vi "Gear.vi"(10 "Gear1?":bool, 11 "Gear0?":bool) -> ()   [LabVIEW 2016]
uses:
  <vilib>/Rock Robotics/WPI/Solenoid/WPI_SolenoidValue.ctl
  <vilib>/Rock Robotics/WPI/Solenoid/WPI_SolenoidSetEnum.vi
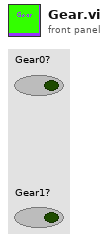
[diagram p1: front panel]
types:
  T1 = typedef "WPI_SolenoidValue.ctl" = enum16{"Off", "On", "Forward", "Reverse"}
  T2 = typedef "WPI_SolenoidDevRef.ctl" = cluster{"DevStatus":errorcluster, "Pneumatics Control Module":u8, "Forward Solenoid Channel":T3, "Reverse Solenoid Channel":T3}
  T3 = typedef "WPI_SolenoidChannel.ctl" = enum8{"Solenoid 0", "Solenoid 1", "Solenoid 2", "Solenoid 3", "Solenoid 4", "Solenoid 5", "Solenoid 6", "Solenoid 7", "Invalid"}
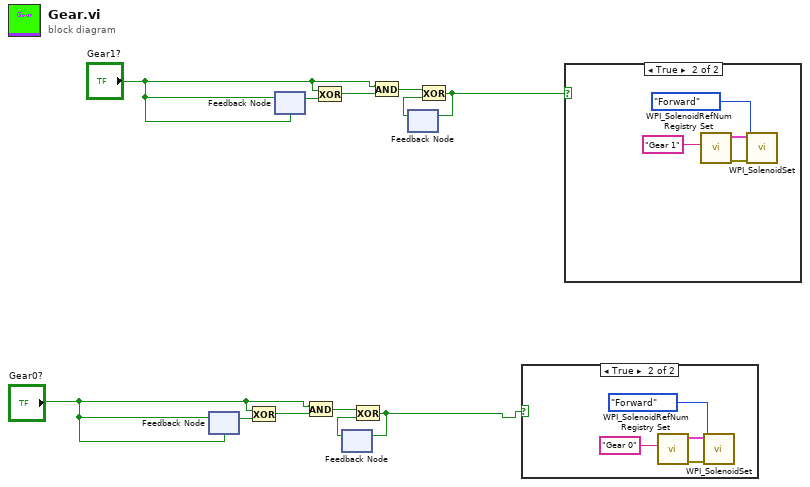
[diagram p0: block diagram]
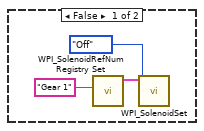
[diagram p2: hidden frame]
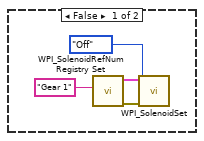
[diagram p3: hidden frame]
diagram:
  n1 = feedback #1("Gear0?") -> (w3:bool)
  n2 = feedback-in #1("Gear0?") -> ()
  n3 = Exclusive Or(1:w3, 2:"Gear0?") -> (0:w4:bool)
  n4 = feedback-in #2("Gear1?") -> ()
  n5 = feedback #2("Gear1?") -> (w12:bool)
  n6 = And(x="Gear0?", y=w4) -> (x .and. y?=w5:bool)
  n7 = Exclusive Or(1:w12, 2:"Gear1?") -> (0:w11:bool)
  n8 = feedback #3() -> (w6:bool)  [unwired: 1 in]
  n9 = Exclusive Or(1:w6, 2:w5) -> (0:w2:bool)
  n10 = feedback-in #3(w2) -> ()
  n11 = And(x="Gear1?", y=w11) -> (x .and. y?=w10:bool)
  n12 = feedback #4() -> (w9:bool)  [unwired: 1 in]
  n13 = Exclusive Or(1:w9, 2:w10) -> (0:w8:bool)
  n14 = feedback-in #4(w8) -> ()
  n15 = case shown="True" w2 {
    frame False {
      n16 = call <vilib>:"WPI_SolenoidRefNum Registry Set.vi"("refnum name"="Gear 1") -> ("SolenoidDevRef"=w15:T2)  [unwired: 9 in, 1 out]
      n17 = call-poly <vilib>:"WPI_SolenoidSet.vi"("Value"=WPI_SolenoidValue."Off", "SolenoidDevRef"=w15) -> ()  [unwired: 8 in, 2 out]
    }
    frame True {
      n18 = call <vilib>:"WPI_SolenoidRefNum Registry Set.vi"("refnum name"="Gear 0") -> ("error out"=w19:errorcluster, "SolenoidDevRef"=w18:T2)  [unwired: 9 in]
      n19 = call-poly <vilib>:"WPI_SolenoidSet.vi"("error in (no error)"=w19, "Value"=WPI_SolenoidValue."Forward", "SolenoidDevRef"=w18) -> ()  [unwired: 7 in, 2 out]
    }
  }
  n20 = case shown="True" w8 {
    frame False {
      n21 = call <vilib>:"WPI_SolenoidRefNum Registry Set.vi"("refnum name"="Gear 1") -> ("error out"=w20:errorcluster, "SolenoidDevRef"=w21:T2)  [unwired: 9 in]
      n22 = call-poly <vilib>:"WPI_SolenoidSet.vi"("error in (no error)"=w20, "Value"=WPI_SolenoidValue."Off", "SolenoidDevRef"=w21) -> ()  [unwired: 7 in, 2 out]
    }
    frame True {
      n23 = call <vilib>:"WPI_SolenoidRefNum Registry Set.vi"("refnum name"="Gear 1") -> ("error out"=w27:errorcluster, "SolenoidDevRef"=w26:T2)  [unwired: 9 in]
      n24 = call-poly <vilib>:"WPI_SolenoidSet.vi"("error in (no error)"=w27, "Value"=WPI_SolenoidValue."Forward", "SolenoidDevRef"=w26) -> ()  [unwired: 7 in, 2 out]
    }
  }
